vi "Start.vi"(8 "error in (no error)":errorcluster, 11 "DAQ Task in":refnum<class "DAQ Task.lvclass">) -> (0 "error out":errorcluster, 3 "DAQ Task out":refnum<class "DAQ Task.lvclass">)   [LabVIEW 2018, in "Data Acquisition.lvlib" / "DAQ Task.lvclass"]
uses:
  DAQ Task.lvclass
  DAQ Task.lvclass/DAQ Task.ctl
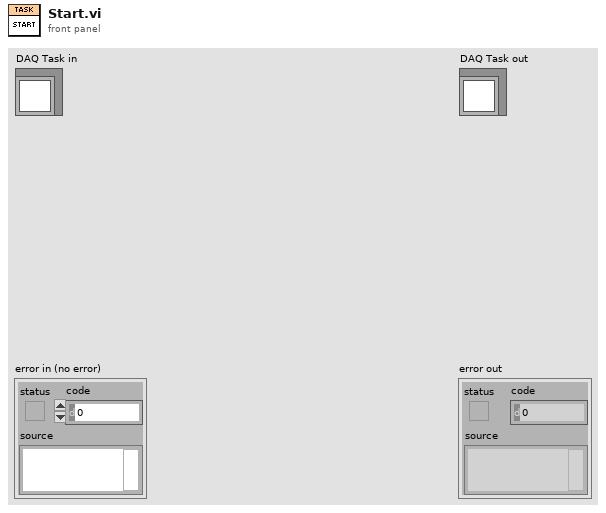
[diagram p1: front panel]
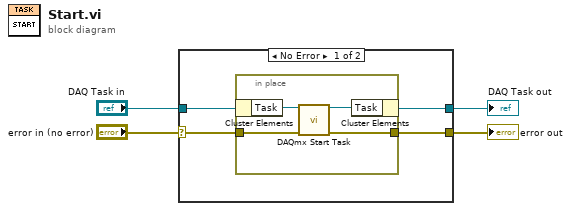
[diagram p0: block diagram]
diagram:
  n1 = case shown="No Error" "error in (no error)" {
    selector: "error in (no error)" -> [w7 w14]
    tunnel: [w6 w14] -> w3
    tunnel: [w5 w13] -> w1
    tunnel: "DAQ Task in" -> [w8 w13]
    frame No Error {
      n2 = in-place {
        in-place-border: w7 -> [w11]
        in-place-border: [w10] -> w6
        n3 = in-place-cluster #1(w8) -> ("Task"=w12:refnum<k21>)
        n4 = call <vilib>:"DAQmx Start Task.vi"("task/channels in"=w12, "error in"=w11) -> ("task out"=w9:refnum<k21>, "error out"=w10:errorcluster)  [unwired: 12 in]
        n5 = in-place-cluster #1("Task"=w9) -> (w5:refnum<class "DAQ Task.lvclass">)
      }
    }
    frame Error {
    }
  }
  "error out" <- w3
  "DAQ Task out" <- w1
